vi "make_request.vi"(8 "Error in":errorcluster, 9 "Accept":string, 10 "Content-Type":string, 11 "Device In":T1) -> (0 "error out":errorcluster, 1 "error":i32, 2 "Comm":T2, 3 "Device Out":T1, 4 "body":string)   [LabVIEW 2019]
uses:
  <userlib>/IoT Devices/_subVIs/HTTPComm.ctl
  <userlib>/Onshape/_SubVI/Cluster.ctl
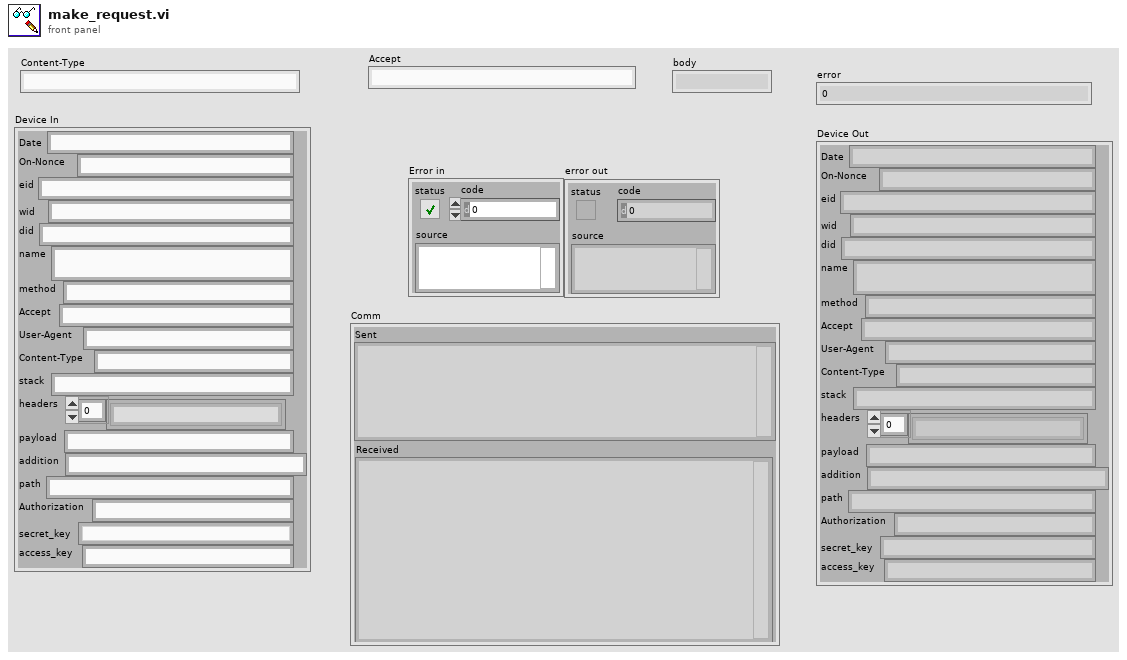
[diagram p1: front panel]
types:
  T1 = typedef "Cluster.ctl" = cluster{"Date":string, "On-Nonce":string, "eid":string, "wid":string, "did":string, "name":string, "method":string, "Accept":string, "User-Agent":string, "Content-Type":string, "stack":string, "headers":string[], "payload":string, "addition":string, "path":string, "Authorization":string, "secret_key":string, "access_key":string}
  T2 = typedef "HTTPComm.ctl" = cluster{"url":string, "sent headers":string, "sent body":string, "headers":string, "body":string, "Sent":string, "Received":string}
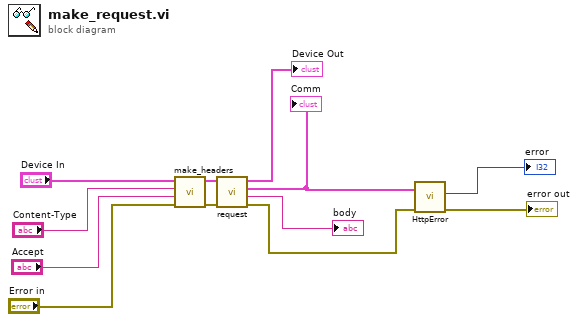
[diagram p0: block diagram]
diagram:
  n1 = call <userlib>:"make_headers.vi"("Error in"="Error in", "Accept"="Accept", "Content-Type"="Content-Type", "Device In"="Device In") -> ("Error Out"=w11:errorcluster, "Device Out"=w12:T1)  [unwired: 6 in]
  n2 = call <userlib>:"request.vi"("Device In"=w12, "error in"=w11) -> ("Device Out"=→"Device Out":T1, "Comm"=w6:T2, "body"=→"body":string, "error out"=w5:errorcluster)  [unwired: 5 in]
  "Comm" <- w6
  n3 = call <userlib>:"HttpError.vi"("error in (no error)"=w5, "Comm"=w6) -> ("error out"=→"error out":errorcluster, "error"=→"error":i32)  [unwired: 8 in]
